vi "Main.vi"() -> ()   [LabVIEW 2010]
uses:
  Control 1.ctl
  DataCluster.ctl
panel:
  in  "結束程式":bool
  in  "倒數計時":bool
  in  "設定鬧鐘":bool
  out "Now":timestamp format="%<%x \n%.X>T"
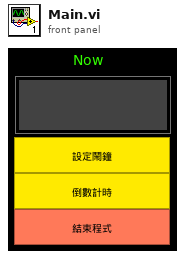
[diagram p1: front panel]
types:
  T1 = typedef "Control 1.ctl" = enum16{"initial", "idle", "set Alarm", "Alarm", "set count down", "CountDown", "End"}
  T2 = typedef "DataCluster.ctl" = cluster{"鬧鐘時間":timestamp, "鈴聲":path, "error ":errorcluster, "Min":dbl, "Sec":dbl, "鬧鐘作用":bool}
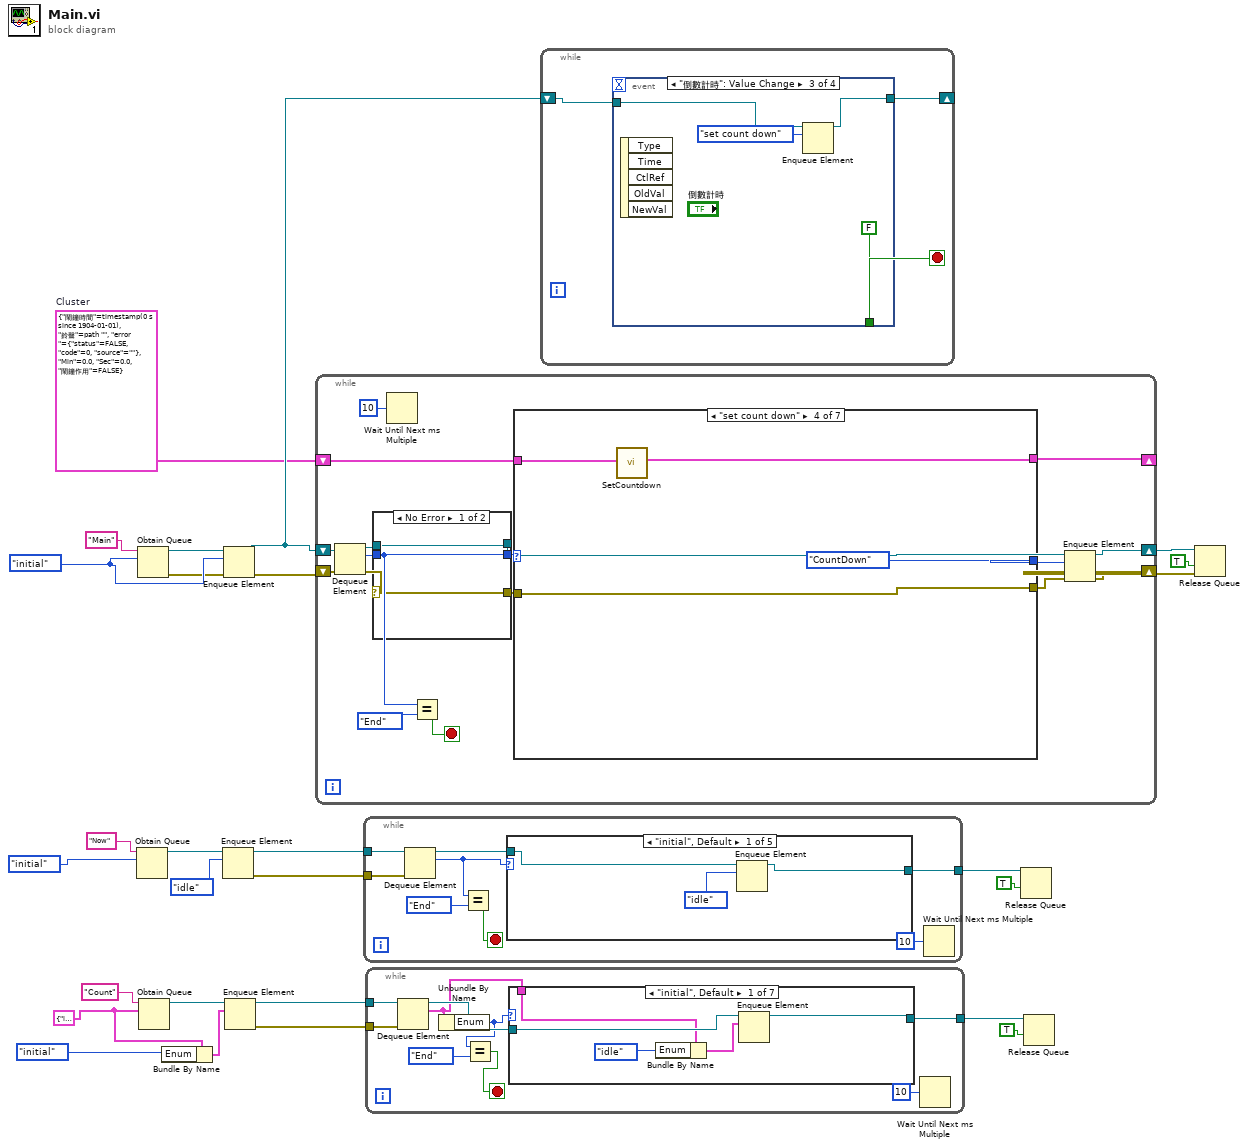
[diagram p0: block diagram]
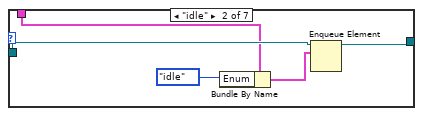
[diagram p2: hidden frame]
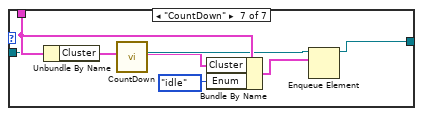
[diagram p7: hidden frame]
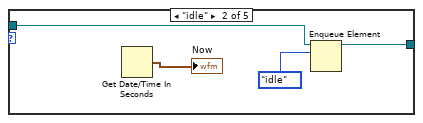
[diagram p8: hidden frame]
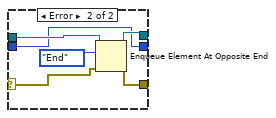
[diagram p12: hidden frame]
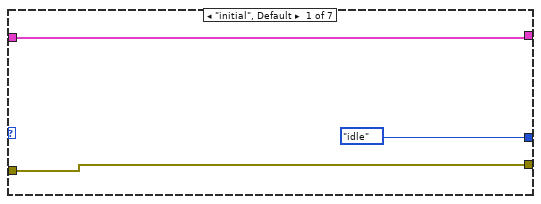
[diagram p13: hidden frame]
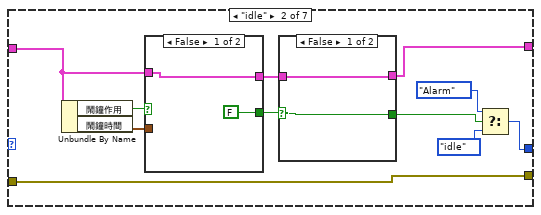
[diagram p14: hidden frame]
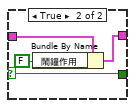
[diagram p15: hidden frame]
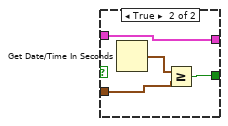
[diagram p16: hidden frame]
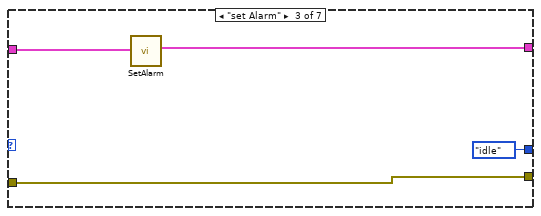
[diagram p17: hidden frame]
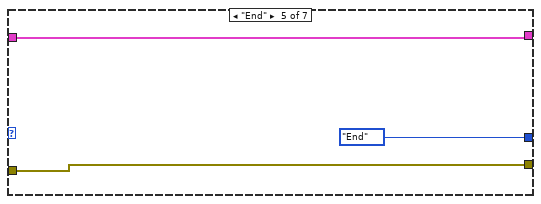
[diagram p18: hidden frame]
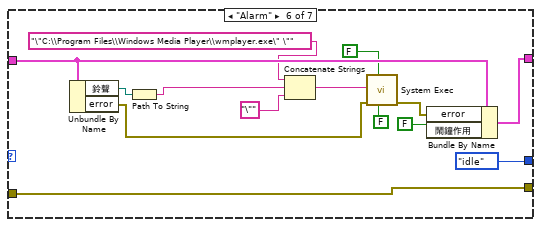
[diagram p19: hidden frame]
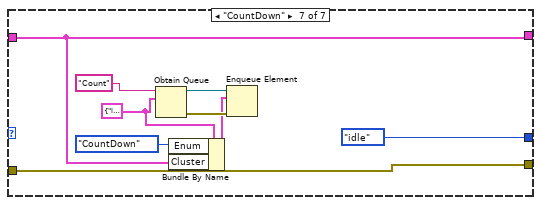
[diagram p20: hidden frame]
diagram:
  w7 = cluster{"Enum":T1, "Cluster":T2} {"Enum"=enum."initial", "Cluster"={"鬧鐘時間"=timestamp(0 s since 1904-01-01), "鈴聲"=path "", "error "={"status"=FALSE, "code"=0, "source"=""}, "Min"=0.0, "Sec"=0.0, "鬧鐘作用"=FALSE}}
  w12 = T2 {"鬧鐘時間"=timestamp(0 s since 1904-01-01), "鈴聲"=path "", "error "={"status"=FALSE, "code"=0, "source"=""}, "Min"=0.0, "Sec"=0.0, "鬧鐘作用"=FALSE}  # Cluster
  w25 = Control_1."initial" ("Enum")
  n1 = Obtain Queue(name (unnamed)="Now", element data type=Control_1."initial" ("Enum")) -> (queue out=w17:refnum<queue>)  [unwired: 3 in, 2 out]
  n2 = Obtain Queue(name (unnamed)="Main", element data type=w25) -> (queue out=w27:refnum<queue>, error out=w24:errorcluster)  [unwired: 3 in, 1 out]
  n3 = Obtain Queue(name (unnamed)="Count", element data type=w7) -> (queue out=w9:refnum<queue>)  [unwired: 3 in, 2 out]
  n4 = Bundle By Name(cluster=w7, "Enum"=Control_1."initial") -> (w5:cluster{"Enum":T1, "Cluster":T2})
  n5 = Enqueue Element(queue=w17, element=Control_1."idle") -> (queue out=w15:refnum<queue>, error out=w14:errorcluster)  [unwired: 2 in, 1 out]
  n6 = Enqueue Element(queue=w27, element=w25, error in (no error)=w24) -> (queue out=w22:refnum<queue>, error out=w23:errorcluster)  [unwired: 1 in, 1 out]
  n7 = Enqueue Element(queue=w9, element=w5) -> (queue out=w10:refnum<queue>, error out=w11:errorcluster)  [unwired: 2 in, 1 out]
  n8 = while {
    shift-right: [w34] -> w19
    shift-left: w23 -> [w42]
    shift-right: [w32] -> w21
    shift-left: w22 -> [w41]
    shift-right: [w28] -> _
    shift-left: w12 -> [w30]
    stop <- w44 stop-if-true
    n9 = Dequeue Element(queue=w41, error in (no error)=w42) -> (queue out=w36:refnum<queue>, element=w39:T1, error out=w40:errorcluster)  [unwired: 1 in, 1 out]
    n10 = case shown="No Error" w40 {
      selector: w40 -> [w46 w51]
      tunnel: w39 -> [w47 w48]
      tunnel: [w47 w48] -> w38
      tunnel: [w46 w50] -> w37
      tunnel: w36 -> [w45 w53]
      tunnel: [w45 w52] -> w33
      frame No Error {
      }
      frame Error {
        n11 = Enqueue Element At Opposite End(queue=w53, element=Control_1."End", error in (no error)=w51) -> (queue out=w52:refnum<queue>, error out=w50:errorcluster)  [unwired: 1 in, 1 out]
      }
    }
    n12 = Wait Until Next ms Multiple(millisecond multiple=u32 10) -> ()  [unwired: 1 out]
    n13 = Equal?(x=w39, y=Control_1."End") -> (x = y?=w44:bool)
    n14 = case shown="\"set count down\"" w38 {
      tunnel: w37 -> [w56 w65 w80 w84 w89 w101 w106]
      tunnel: [w56 w65 w80 w84 w89 w101 w106] -> w35
      tunnel: [Control_1."idle" ("element") w66 Control_1."idle" ("element") Control_1."CountDown" ("element") Control_1."End" ("element") Control_1."idle" ("element") Control_1."idle" ("element")] -> w31
      tunnel: w30 -> [w54 w61 w83 w87 w90 w104 w105]
      tunnel: [w54 w58 w82 w86 w90 w103 w105] -> w28
      frame "initial", Default {
      }
      frame "idle" {
        n15 = Unbundle By Name(w61) -> ("鬧鐘作用"=w63:bool, "鬧鐘時間"=w62:timestamp)
        n16 = case shown="False" w63 {
          tunnel: [FALSE w78] -> w60
          tunnel: w62 -> [_ w77]
          tunnel: w61 -> [w74 w76]
          tunnel: [w74 w76] -> w59
          frame False {
          }
          frame True {
            n17 = Get Date/Time In Seconds() -> (seconds since 1Jan1904=w79:timestamp)
            n18 = Greater Or Equal?(x=w79, y=w77) -> (x >= y?=w78:bool)
          }
        }
        n19 = case shown="False" w60 {
          selector: w60 -> [w68 w70]
          tunnel: w59 -> [w69 w73]
          tunnel: [w69 w71] -> w58
          tunnel: [w68 w70] -> w57
          frame False {
          }
          frame True {
            n20 = Bundle By Name(cluster=w73, "鬧鐘作用"=FALSE) -> (w71:T2)
          }
        }
        n21 = Select(t=Control_1."Alarm" ("Enum"), s=w57, f=Control_1."idle" ("Enum")) -> (s? t:f=w66:T1)
      }
      frame "set Alarm" {
        n22 = call "SetAlarm.vi"("Cluster 2"=w83) -> ("Cluster"=w82:T2)  [unwired: 10 in]
      }
      frame "set count down" {
        n23 = call "SetCountdown.vi"("Cluster 2"=w87) -> ("Cluster"=w86:T2)  [unwired: 10 in]
      }
      frame "End" {
      }
      frame "Alarm" {
        n24 = Unbundle By Name(w104) -> ("鈴聲"=w96:path, "error"=w92:errorcluster)
        n25 = Path To String(path=w96) -> (string=w98:string)
        n26 = Concatenate Strings("\"C:\\Program Files\\Windows Media Player\\wmplayer.exe\" \"" ("command line"), w98, "\"" ("string")) -> (w99:string)
        n27 = call <vilib>:"System Exec.vi"("run minimized? (F)"=FALSE, "wait until completion? (T)"=FALSE, "error in (no error)"=w92, "command line"=w99) -> ("error out"=w91:errorcluster)  [unwired: 4 in, 3 out]
        n28 = Bundle By Name(cluster=w104, "error"=w91, "鬧鐘作用"=FALSE) -> (w103:T2)
      }
      frame "CountDown" {
        w108 = cluster{"Enum":T1, "Cluster":T2} {"Enum"=enum."initial", "Cluster"={"鬧鐘時間"=timestamp(0 s since 1904-01-01), "鈴聲"=path "", "error "={"status"=FALSE, "code"=0, "source"=""}, "Min"=0.0, "Sec"=0.0, "鬧鐘作用"=FALSE}}
        n29 = Obtain Queue(name (unnamed)="Count", element data type=w108) -> (queue out=w112:refnum<queue>, error out=w111:errorcluster)  [unwired: 3 in, 1 out]
        n30 = Bundle By Name(cluster=w108, "Enum"=Control_1."CountDown", "Cluster"=w105) -> (w109:cluster{"Enum":T1, "Cluster":T2})
        n31 = Enqueue Element(queue=w112, element=w109, error in (no error)=w111) -> ()  [unwired: 1 in, 3 out]
      }
    }
    n32 = Enqueue Element(queue=w33, element=w31, error in (no error)=w35) -> (queue out=w32:refnum<queue>, error out=w34:errorcluster)  [unwired: 1 in, 1 out]
  }
  n33 = while {
    tunnel: w15 -> [w121]
    tunnel: w14 -> [w120]
    tunnel: [w114] -> w3
    stop <- w116 stop-if-true
    n34 = Dequeue Element(queue=w121, error in (no error)=w120) -> (queue out=w119:refnum<queue>, element=w118:T1)  [unwired: 1 in, 2 out]
    n35 = Equal?(x=w118, y=Control_1."End") -> (x = y?=w116:bool)
    n36 = case shown="\"initial\", Default" w118 {
      tunnel: w119 -> [w123 w126 _ _ w129]
      tunnel: [w122 w125 _ _ w129] -> w114
      frame "initial", Default {
        n37 = Enqueue Element(queue=w123, element=Control_1."idle") -> (queue out=w122:refnum<queue>)  [unwired: 2 in, 2 out]
      }
      frame "idle" {
        n38 = Get Date/Time In Seconds() -> (seconds since 1Jan1904=→"Now":timestamp)
        n39 = Enqueue Element(queue=w126, element=Control_1."idle") -> (queue out=w125:refnum<queue>)  [unwired: 2 in, 2 out]
      }
      frame "set Alarm" {
      }
      frame "set count down" {
      }
      frame "End" {
      }
    }
    n40 = Wait Until Next ms Multiple(millisecond multiple=u32 10) -> ()  [unwired: 1 out]
  }
  n41 = while {
    tunnel: w10 -> [w138]
    tunnel: w11 -> [w137]
    tunnel: [w130] -> w1
    stop <- w132 stop-if-true
    n42 = Dequeue Element(queue=w138, error in (no error)=w137) -> (queue out=w136:refnum<queue>, element=w133:cluster{"Enum":T1, "Cluster":T2})  [unwired: 1 in, 2 out]
    n43 = Unbundle By Name(w133) -> ("Enum"=w134:T1)
    n44 = Equal?(x=w134, y=Control_1."End") -> (x = y?=w132:bool)
    n45 = case shown="\"initial\", Default" w134 {
      tunnel: w136 -> [w143 w148 w149 w150 w151 w152 w155]
      tunnel: w133 -> [w142 w147 _ _ _ _ w158]
      tunnel: [w139 w144 w149 w150 w151 w152 w153] -> w130
      frame "initial", Default {
        n46 = Bundle By Name(cluster=w142, "Enum"=Control_1."idle" ("element")) -> (w140:cluster{"Enum":T1, "Cluster":T2})
        n47 = Enqueue Element(queue=w143, element=w140) -> (queue out=w139:refnum<queue>)  [unwired: 2 in, 2 out]
      }
      frame "idle" {
        n48 = Bundle By Name(cluster=w147, "Enum"=Control_1."idle" ("element")) -> (w145:cluster{"Enum":T1, "Cluster":T2})
        n49 = Enqueue Element(queue=w148, element=w145) -> (queue out=w144:refnum<queue>)  [unwired: 2 in, 2 out]
      }
      frame "set Alarm" {
      }
      frame "set count down" {
      }
      frame "End" {
      }
      frame "Alarm" {
      }
      frame "CountDown" {
        n50 = Unbundle By Name(w158) -> ("Cluster"=w159:T2)
        n51 = call "CountDown.vi"("Cluster"=w159) -> ("Cluster 2"=w154:T2)  [unwired: 10 in]
        n52 = Bundle By Name(cluster=w158, "Cluster"=w154, "Enum"=Control_1."idle" ("element")) -> (w156:cluster{"Enum":T1, "Cluster":T2})
        n53 = Enqueue Element(queue=w155, element=w156) -> (queue out=w153:refnum<queue>)  [unwired: 2 in, 2 out]
      }
    }
    n54 = Wait Until Next ms Multiple(millisecond multiple=u32 10) -> ()  [unwired: 1 out]
  }
  n55 = while {
    shift-right: [w160] -> _
    shift-left: w22 -> [w162]
    stop <- w161 stop-if-true
    n56 = event shown="[2] \"倒數計時\": Value Change" {
      selector: _ -> [_ _ _ _]
      dyn-events: _ -> [_ _ _ _]
      timeout: _ -> [_ _ _ _]
      tunnel: w162 -> [_ w165 w170 _]
      tunnel: [_ FALSE FALSE TRUE] -> w161
      tunnel: [_ w163 w168 _] -> w160
      event Timeout {
        n57 = event-data() -> ()  [unwired: 1 in, 2 out]
      }
      event "設定鬧鐘": Value Change {
        n58 = event-data() -> ()  [unwired: 1 in, 5 out]
        n59 = Enqueue Element(queue=w165, element=Control_1."set Alarm") -> (queue out=w163:refnum<queue>)  [unwired: 2 in, 2 out]
      }
      event "倒數計時": Value Change {
        n60 = event-data() -> ()  [unwired: 1 in, 5 out]
        n61 = Enqueue Element(queue=w170, element=Control_1."set count down") -> (queue out=w168:refnum<queue>)  [unwired: 2 in, 2 out]
      }
      event "結束程式": Value Change {
        w174 = cluster{"Enum":T1, "Cluster":T2} {"Enum"=enum."initial", "Cluster"={"鬧鐘時間"=timestamp(0 s since 1904-01-01), "鈴聲"=path "", "error "={"status"=FALSE, "code"=0, "source"=""}, "Min"=0.0, "Sec"=0.0, "鬧鐘作用"=FALSE}}
        w177 = Control_1."End" ("element")
        n62 = event-data() -> ()  [unwired: 1 in, 5 out]
        n63 = Obtain Queue(name (unnamed)="Main", element data type=w177) -> (queue out=w180:refnum<queue>)  [unwired: 3 in, 2 out]
        n64 = Obtain Queue(name (unnamed)="Now", element data type=w177) -> (queue out=w179:refnum<queue>)  [unwired: 3 in, 2 out]
        n65 = Obtain Queue(name (unnamed)="Count", element data type=w174) -> (queue out=w171:refnum<queue>)  [unwired: 3 in, 2 out]
        n66 = Bundle By Name(cluster=w174, "Enum"=Control_1."End") -> (w172:cluster{"Enum":T1, "Cluster":T2})
        n67 = Enqueue Element(queue=w180, element=w177) -> ()  [unwired: 2 in, 3 out]
        n68 = Enqueue Element(queue=w179, element=w177) -> ()  [unwired: 2 in, 3 out]
        n69 = Enqueue Element(queue=w171, element=w172) -> ()  [unwired: 2 in, 3 out]
      }
    }
  }
  n70 = Release Queue(queue=w3, force destroy? (F)=TRUE) -> ()  [unwired: 1 in, 3 out]
  n71 = Release Queue(queue=w1, force destroy? (F)=TRUE) -> ()  [unwired: 1 in, 3 out]
  n72 = Release Queue(queue=w21, force destroy? (F)=TRUE, error in (no error)=w19) -> ()  [unwired: 3 out]
